vi "lab1.vi"() -> ()   [LabVIEW 2013]
panel:
  in  "stop":bool
  out "Array":bool[](array[boolean])
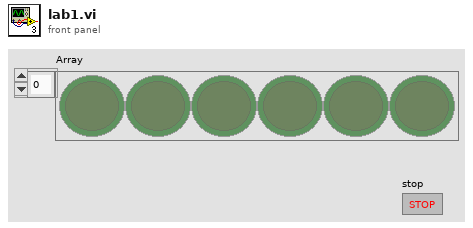
[diagram p1: front panel]
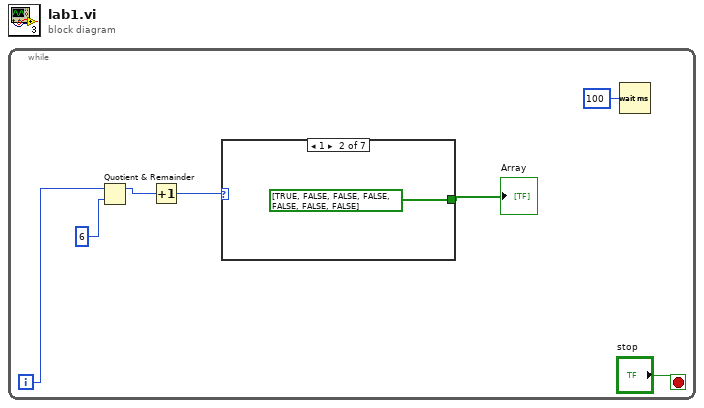
[diagram p0: block diagram]
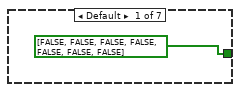
[diagram p2: hidden frame]
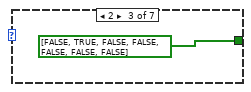
[diagram p3: hidden frame]
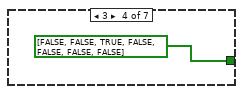
[diagram p4: hidden frame]
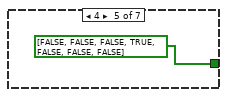
[diagram p5: hidden frame]
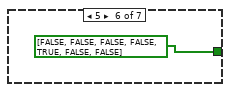
[diagram p6: hidden frame]
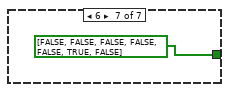
[diagram p7: hidden frame]
diagram:
  n1 = while {
    i -> [w6]
    stop <- "stop" stop-if-true
    n2 = Quotient & Remainder(x=w6, y=6) -> (x-y*floor(x/y)=w4:i32)  [unwired: 1 out]
    n3 = Increment(x=w4) -> (x+1=w3:i32)
    n4 = case shown="1" w3 {
      tunnel: [bool[] [FALSE, FALSE, FALSE, FALSE, FALSE, FALSE, FALSE] bool[] [TRUE, FALSE, FALSE, FALSE, FALSE, FALSE, FALSE] bool[] [FALSE, TRUE, FALSE, FALSE, FALSE, FALSE, FALSE] bool[] [FALSE, FALSE, TRUE, FALSE, FALSE, FALSE, FALSE] bool[] [FALSE, FALSE, FALSE, TRUE, FALSE, FALSE, FALSE] bool[] [FALSE, FALSE, FALSE, FALSE, TRUE, FALSE, FALSE] bool[] [FALSE, FALSE, FALSE, FALSE, FALSE, TRUE, FALSE]] -> w7
      frame Default {
      }
      frame 1 {
      }
      frame 2 {
      }
      frame 3 {
      }
      frame 4 {
      }
      frame 5 {
      }
      frame 6 {
      }
    }
    "Array" <- w7
    n5 = Wait (ms)(milliseconds to wait=u32 100) -> ()  [unwired: 1 out]
  }
